vi "find all files withing a folder.vi"(0 "folders":cluster{"file path":path, "depth":i32}[](array[cluster])) -> (1 "filenames":string[](array[string]), 2 "paths":path[](array[path]))   [LabVIEW 2009]
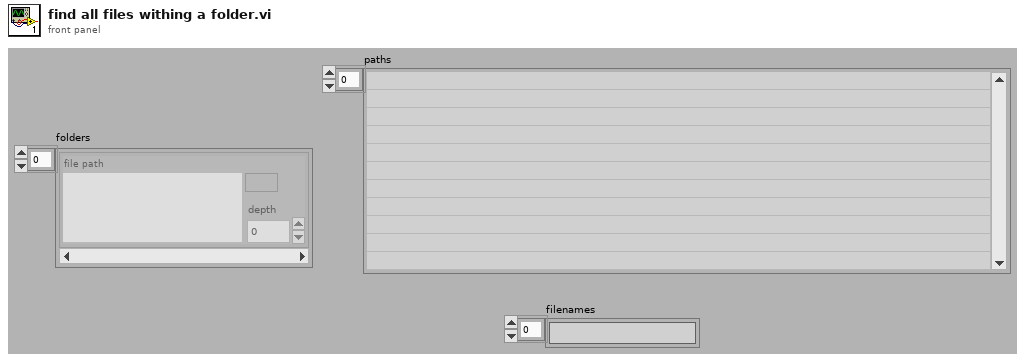
[diagram p1: front panel]
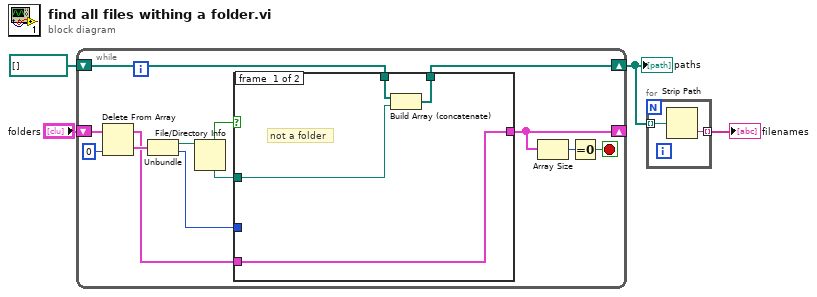
[diagram p0: block diagram]
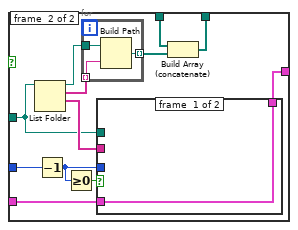
[diagram p2: hidden frame]
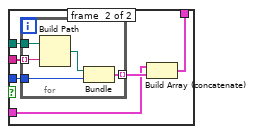
[diagram p3: hidden frame]
diagram:
  n1 = while {
    shift-right: [w6] -> _
    shift-left: "folders" -> [w13]
    shift-right: [w14] -> w2
    shift-left: path[] [] -> [w15]
    stop <- w9 stop-if-true
    n2 = Delete From Array(array=w13, index=0) -> (deleted portion=w16:cluster{"file path":path, "depth":i32}, array with subset deleted=w11:cluster{"file path":path, "depth":i32}[])  [unwired: 1 in]
    n3 = Unbundle(w16) -> ("file path"=w8:path, "depth"=w17:i32)
    n4 = File/Directory Info(path=w8) -> (directory=w5:bool, resolved path=w7:path)  [unwired: 1 in, 5 out]
    n5 = case shown="True" w5 {
      tunnel: w17 -> [_ w30]
      tunnel: w15 -> [w20 w28]
      tunnel: [w21 w27] -> w14
      tunnel: w11 -> [w18 w24]
      tunnel: [w18 w23] -> w6
      tunnel: w7 -> [w19 w22]
      frame #0 {
        # "not a folder"
        n6 = Build Array (concatenate)(w20, w19) -> (w21:path[])
      }
      frame #1 {
        n7 = List Folder(path=w22) -> (path out=w33:path, filenames=w32:string[], folder names=w31:string[])  [unwired: 3 in, 1 out]
        n8 = Decrement(x=w30) -> (x-1=w26:i32)
        n9 = Greater Or Equal To 0?(x=w26) -> (x >= 0?=w25:bool)
        n10 = for {
          tunnel: w32 -> [w47] mode=indexing
          tunnel: w33 -> [w48]
          tunnel: [w46] -> w29 mode=indexing
          n11 = Build Path(base path=w48, name or relative path=w47) -> (appended path=w46:path)
        }
        n12 = case shown="True" w25 {
          tunnel: w31 -> [_ w40]
          tunnel: w22 -> [_ w39]
          tunnel: w24 -> [w34 w37]
          tunnel: [w34 w36] -> w23
          tunnel: w26 -> [_ w35]
          frame #0 {
          }
          frame #1 {
            n13 = for {
              tunnel: w40 -> [w44] mode=indexing
              tunnel: w39 -> [w45]
              tunnel: w35 -> [w42]
              tunnel: [w41] -> w38 mode=indexing
              n14 = Build Path(base path=w45, name or relative path=w44) -> (appended path=w43:path)
              n15 = Bundle("appended path"=w43, w42) -> (w41:cluster{"appended path":path, i32})  [unwired: 1 in]
            }
            n16 = Build Array (concatenate)(w37, w38) -> (w36:cluster{"appended path":path, "depth":i32}[])
          }
        }
        n17 = Build Array (concatenate)(w28, w29) -> (w27:path[])
      }
    }
    n18 = Array Size(array=w6) -> (size(s)=w10:i32)
    n19 = Equal To 0?(x=w10) -> (x = 0?=w9:bool)
  }
  "paths" <- w2
  n20 = for {
    tunnel: w2 -> [w50] mode=indexing
    tunnel: [w49] -> w1 mode=indexing
    n21 = Strip Path(path=w50) -> (name=w49:string)  [unwired: 1 out]
  }
  "filenames" <- w1
